vi "2.3.vi"() -> ()   [LabVIEW 2020]
panel:
  out "Temp a 90 °":bool
  out "Estado":string
  out "Thermometer":dbl(slide) scale=0.0..100.0
  in  "stop":bool
  out "Waveform Chart":i32(graph)
  out "Indicador":dbl
  out "Tanque FULL":bool
  out "Tanque lleno a la mitad":bool
  out "Tanque vacio":bool
  out "Tank":dbl(slide) scale=0.0..100.0
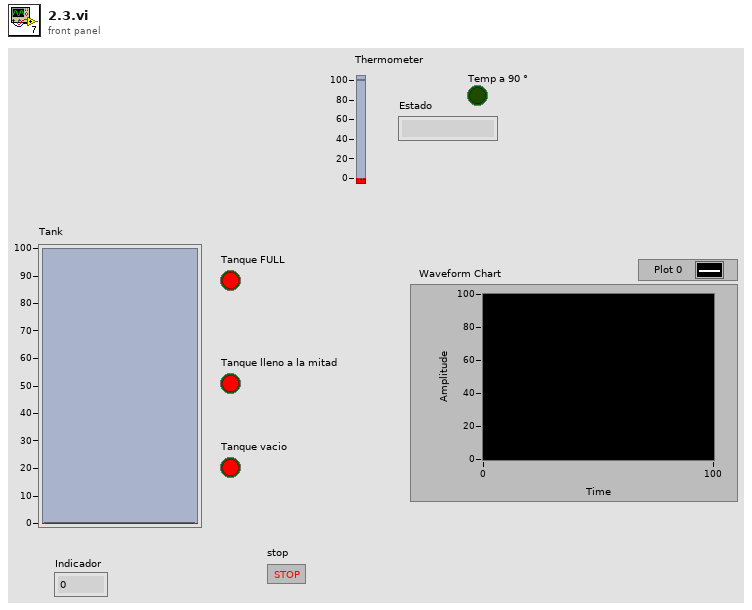
[diagram p1: front panel]
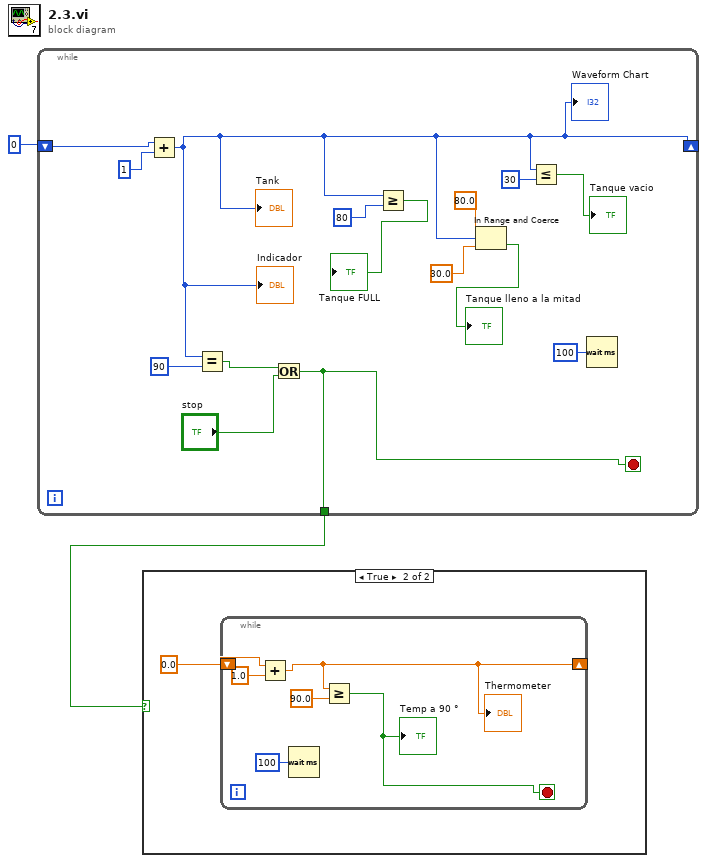
[diagram p0: block diagram]
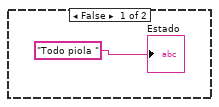
[diagram p2: hidden frame]
diagram:
  n1 = while {
    shift-right: [w6] -> _
    shift-left: 0 -> [w17]
    tunnel: [w3] -> w1
    stop <- w3 stop-if-true
    n2 = Add(x=w17, y=1) -> (x+y=w6:i32)
    "Tank" <- w6
    "Indicador" <- w6
    "Waveform Chart" <- w6
    n3 = Equal?(x=w6, y=90) -> (x = y?=w4:bool)
    n4 = Or(x=w4, y="stop") -> (x .or. y?=w3:bool)
    n5 = Greater Or Equal?(x=w6, y=80) -> (x >= y?=→"Tanque FULL":bool)
    n6 = In Range and Coerce(upper limit=80.0, x=w6, lower limit=30.0) -> (In Range?=→"Tanque lleno a la mitad":bool)  [unwired: 1 out]
    n7 = Less Or Equal?(x=w6, y=30) -> (x <= y?=→"Tanque vacio":bool)
    n8 = Wait (ms)(milliseconds to wait=u32 100) -> ()  [unwired: 1 out]
  }
  n9 = case shown="True" w1 {
    frame False {
      "Estado" <- "Todo piola "
    }
    frame True {
      n10 = while {
        shift-right: [w23] -> _
        shift-left: 0.0 -> [w25]
        stop <- w21 stop-if-true
        n11 = Add(x=w25, y=1.0) -> (x+y=w23:dbl)
        "Thermometer" <- w23
        n12 = Wait (ms)(milliseconds to wait=u32 100) -> ()  [unwired: 1 out]
        n13 = Greater Or Equal?(x=w23, y=90.0) -> (x >= y?=w21:bool)
        "Temp a 90 °" <- w21
      }
    }
  }
